vi "init_data_in.vi"(8 "error in (no error)":errorcluster, 11 "input channel":tag) -> (0 "error out":errorcluster, 3 "task out":refnum<k24>)   [LabVIEW 2015]
uses:
  <vilib>/ULx/Create Channel.llb/ULx Create Channel (AI-Voltage-Basic).vi
  C:/Program Files/National Instruments/LabVIEW 2015/vi.lib/ULx/ULx_LV.dll
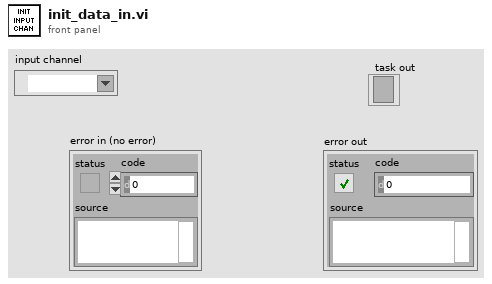
[diagram p1: front panel]
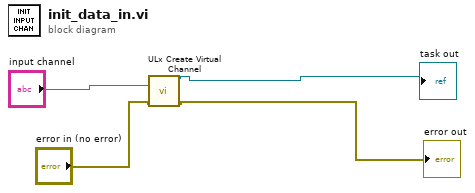
[diagram p0: block diagram]
diagram:
  n1 = call-poly <vilib>:"ULx Create Virtual Channel.vi"("physical channels"="input channel", "error in"="error in (no error)") -> ("task out"=→"task out":refnum<k24>, "error out"=→"error out":errorcluster)  [unwired: 12 in]
